vi "SP Adjust Limit Wavform to Most Constrictive.vi"(6 "Pass?":bool, 7 "Waveforms In":waveform(dbl)[](array[waveform]), 8 "error in (no error)":errorcluster, 9 "Waveform In":waveform(dbl), 10 "Channel Name":string, 11 "Attribute Name (NI_ChannelName)":string) -> (0 "error out":errorcluster, 5 "Waveforms Out":waveform(dbl)[](array[waveform]))   [LabVIEW 2011]
uses:
  Channel Test Status Enumeration.ctl
  TypeDefs/SP Channel Type.ctl
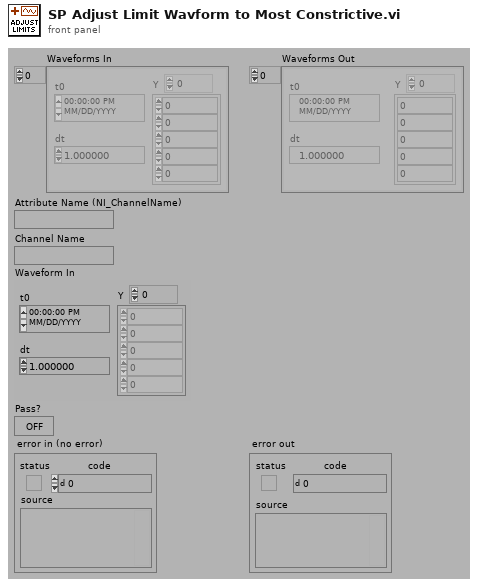
[diagram p1: front panel]
types:
  T1 = typedef "SP Channel Type.ctl" = enum16{"Frequency", "Data", "Limit", "Adapter", "Memory", "Value", "Value Limit"}
  T2 = typedef "Channel Test Status Enumeration.ctl" = enum16{"Fail", "Pass", "Abort", "Error", "Done", "Pass by Sample", "Fail by Sample", "Pass Override", "Fail Override", "Not Tested"}
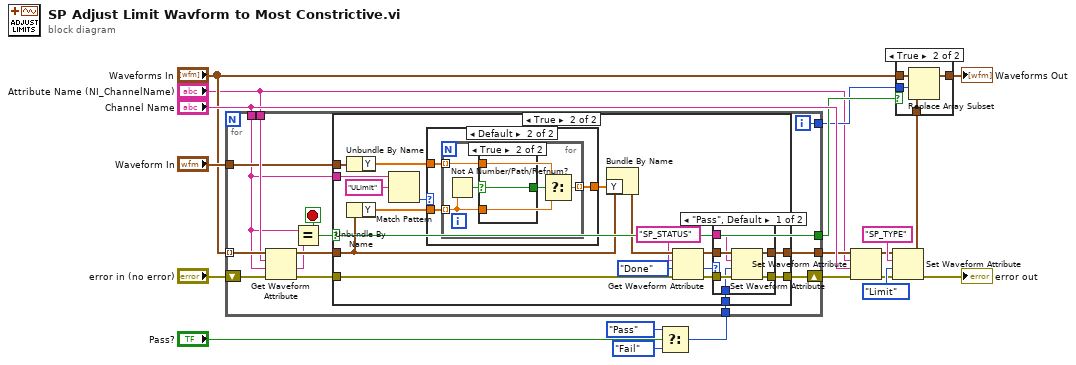
[diagram p0: block diagram]
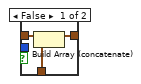
[diagram p2: hidden frame]
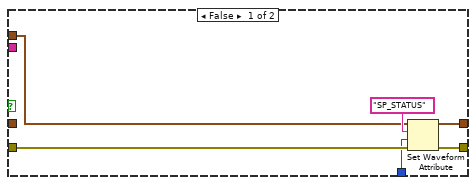
[diagram p3: hidden frame]
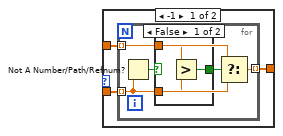
[diagram p5: hidden frame]
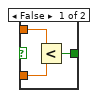
[diagram p7: hidden frame]
diagram:
  n1 = Select(t=Channel_Test_Status_Enumeration."Pass" ("Channel Status Enumeration"), s="Pass?", f=Channel_Test_Status_Enumeration."Fail" ("Channel Status Enumeration")) -> (s? t:f=w3:T2)
  n2 = for {
    tunnel: "Waveforms In" -> [w32] mode=indexing
    shift-right: [w22] -> w16
    shift-left: "error in (no error)" -> [w33]
    tunnel: "Attribute Name (NI_ChannelName)" -> [w31]
    tunnel: "Channel Name" -> [w26]
    tunnel: "Waveform In" -> [w29]
    tunnel: [w28] -> w13
    tunnel: [w24] -> w12
    tunnel: [w27] -> w11
    tunnel: w3 -> [w21]
    i -> [w27]
    stop <- w24 stop-if-true
    n3 = Get Waveform Attribute(4:w33, 5:w26, 6:w31, 7:w32) -> (0:w23:errorcluster, 1:w25:string, 3:w30:waveform(dbl))  [unwired: 1 out]
    n4 = Equal?(x=w26, y=w25) -> (x = y?=w24:bool)
    n5 = case shown="True" w24 {
      tunnel: w30 -> [_ w49]
      tunnel: w26 -> [_ w57]
      tunnel: w29 -> [w35 w53]
      tunnel: [w38 w42] -> w28
      tunnel: w23 -> [w36 w50]
      tunnel: [w37 w41] -> w22
      tunnel: w21 -> [w34 w40]
      frame False {
        n6 = Set Waveform Attribute(4:w36, 5:w34, 6:"SP_STATUS", 7:w35) -> (0:w37:errorcluster, 3:w38:waveform(dbl))  [unwired: 1 out]
      }
      frame True {
        w43 = "SP_STATUS"
        n7 = Unbundle By Name(w53) -> ("Y"=w52:dbl[])
        n8 = Unbundle By Name(w49) -> ("Y"=w54:dbl[])
        n9 = Match Pattern(string=w57, regular expression="ULimit") -> (offset past match=w55:i32)  [unwired: 4 out]
        n10 = case shown="Default" w55 {
          tunnel: w54 -> [w67 w79]
          tunnel: w52 -> [w66 w80]
          tunnel: [w68 w78] -> w51
          frame -1 {
            n11 = for {
              tunnel: w67 -> [w70] mode=indexing
              tunnel: w66 -> [w72] mode=indexing
              tunnel: [w71] -> w68 mode=indexing
              n12 = Not A Number/Path/Refnum?(number/path/refnum=w70) -> (NaN/Path/Refnum?=w69:bool)
              n13 = case shown="False" w69 {
                selector: w69 -> [_ w77]
                tunnel: [w76 w77] -> w73
                tunnel: w72 -> [w75 _]
                tunnel: w70 -> [w74 _]
                frame False {
                  n14 = Greater?(x=w75, y=w74) -> (0:w76:bool)
                }
                frame True {
                }
              }
              n15 = Select(t=w72, s=w73, f=w70) -> (s? t:f=w71:dbl)
            }
          }
          frame Default {
            n16 = for {
              tunnel: w79 -> [w82] mode=indexing
              tunnel: w80 -> [w84] mode=indexing
              tunnel: [w83] -> w78 mode=indexing
              n17 = Not A Number/Path/Refnum?(number/path/refnum=w82) -> (NaN/Path/Refnum?=w81:bool)
              n18 = case shown="True" w81 {
                selector: w81 -> [_ w89]
                tunnel: [w88 w89] -> w85
                tunnel: w84 -> [w87 _]
                tunnel: w82 -> [w86 _]
                frame False {
                  n19 = Less?(x=w87, y=w86) -> (x < y?=w88:bool)
                }
                frame True {
                }
              }
              n20 = Select(t=w84, s=w85, f=w82) -> (s? t:f=w83:dbl)
            }
          }
        }
        n21 = Bundle By Name(cluster=w49, "Y"=w51) -> (w48:waveform(dbl))
        n22 = Get Waveform Attribute(4:w50, 5:Channel_Test_Status_Enumeration."Done" ("Channel Status Enumeration"), 6:w43, 7:w48) -> (0:w44:errorcluster, 1:w46:T2, 3:w45:waveform(dbl))  [unwired: 1 out]
        n23 = case shown="\"Pass\", Default" w46 {
          tunnel: w45 -> [w62 w65]
          tunnel: w44 -> [w63 w64]
          tunnel: w43 -> [w61 _]
          tunnel: [w60 w65] -> w42
          tunnel: [w59 w64] -> w41
          tunnel: w40 -> [w58 _]
          frame "Pass", Default {
            n24 = Set Waveform Attribute(4:w63, 5:w58, 6:w61, 7:w62) -> (0:w59:errorcluster, 3:w60:waveform(dbl))  [unwired: 1 out]
          }
          frame "Fail" {
          }
        }
      }
    }
  }
  n25 = Set Waveform Attribute(4:w16, 5:"Channel Name", 6:"Attribute Name (NI_ChannelName)", 7:w13) -> (0:w1:errorcluster, 3:w2:waveform(dbl))  [unwired: 1 out]
  n26 = Set Waveform Attribute(4:w1, 5:SP_Channel_Type."Limit" ("Channel Type"), 6:"SP_TYPE", 7:w2) -> (0:→"error out":errorcluster, 3:w7:waveform(dbl))  [unwired: 1 out]
  n27 = case shown="True" w12 {
    tunnel: w11 -> [_ w96]
    tunnel: "Waveforms In" -> [w92 w95]
    tunnel: [w91 w94] -> w9
    tunnel: w7 -> [w90 w93]
    frame False {
      n28 = Build Array (concatenate)(w92, w90) -> (w91:waveform(dbl)[])
    }
    frame True {
      n29 = Replace Array Subset(array=w95, new element=w93, index=w96) -> (w94:waveform(dbl)[])
    }
  }
  "Waveforms Out" <- w9
